vi "onPublish.vi"(8 "error in (no error)":errorcluster, 10 "PUBLISH":refnum<class "PUBLISH.lvclass">, 11 "Client in":refnum<class "Client.lvclass">) -> (0 "error out":errorcluster, 3 "Client out":refnum<class "Client.lvclass">)   [LabVIEW 2013, in "MQTT Server.lvlib" / "Client.lvclass"]
uses:
  Client.lvclass
  Control Packets/PUBLISH/PUBLISH.lvclass
  Client.lvclass/Client.ctl
  Server/Session/Session.lvclass
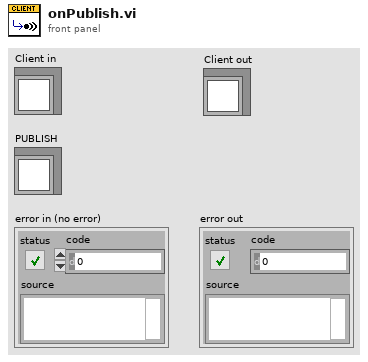
[diagram p1: front panel]
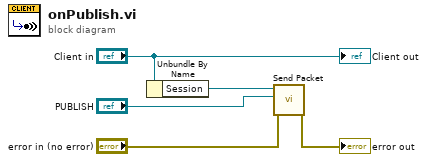
[diagram p0: block diagram]
diagram:
  n1 = Unbundle By Name("Client in") -> ("Session"=w2:refnum<class "Session.lvclass">)
  n2 = call "Send Packet.vi"("error in (no error)"="error in (no error)", "Packet"="PUBLISH", "Session in"=w2) -> ("error out"=→"error out":errorcluster)  [unwired: 6 in, 2 out]
  "Client out" <- "Client in"
